vi "test-vi-1.vi"() -> ()   [LabVIEW 2016, in "test-Application.lvlib"]
uses:
  test-Application.lvlib
panel:
  in  "test-ctl":dbl
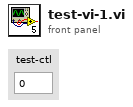
[diagram p1: front panel]
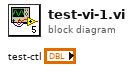
[diagram p0: block diagram]
diagram:
